vi "MatrixDUTSwitch.vi"(8 "error in (no error)":errorcluster, 10 "Channel #":string, 11 "KE3700A in":refnum<class "KE3706A.lvclass">) -> (0 "error out":errorcluster, 3 "KE3700A out":refnum<class "KE3706A.lvclass">)   [LabVIEW 2013, in "KE3706A.lvclass"]
uses:
  KE3706A.lvclass
  <instrlib>/Keithley 3706/Keithley 3700 Series.lvlib
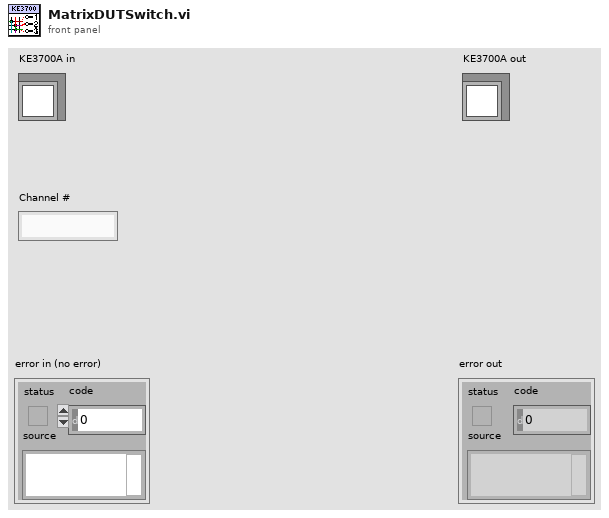
[diagram p1: front panel]
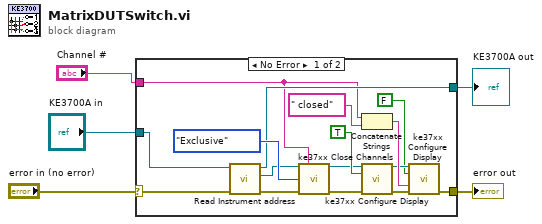
[diagram p0: block diagram]
diagram:
  n1 = case shown="No Error" "error in (no error)" {
    selector: "error in (no error)" -> [w19 w23]
    tunnel: [w7 w23] -> w4
    tunnel: "KE3700A in" -> [w20 w22]
    tunnel: [w16 w22] -> w2
    tunnel: "Channel #" -> [w6 _]
    frame No Error {
      n2 = call-dynamic "Read Instrument address.vi"("error in (no error)"=w19, "InstControl in"=w20) -> ("error out"=w18:errorcluster, "GPIB address"=w17:refnum<visa-resource-name>, "InstControl out"=w16:refnum<class "KE3706A.lvclass">)  [unwired: 7 in]
      n3 = call <instrlib>:"ke37xx Close Channels.vi"("VISA Resource Name"=w17, "Channel List"=w6, "Mode (0: Normal)"=enum16{"Normal", "Exclusive", "Slot Exclusive"}."Exclusive", "error in (no error)"=w18) -> ("VISA Resource Name Out"=w9:refnum<visa-resource-name>, "error out"=w8:errorcluster)  [unwired: 10 in]
      n4 = Concatenate Strings(w6, " closed") -> (w15:string)
      n5 = call <instrlib>:"ke37xx Configure Display.vi"("VISA Resource Name"=w9, "Clear Display (False)"=TRUE, "error in (no error)"=w8) -> ("VISA Resource Name Out"=w13:refnum<visa-resource-name>, "error out"=w10:errorcluster)  [unwired: 11 in]
      n6 = call <instrlib>:"ke37xx Configure Display.vi"("VISA Resource Name"=w13, "Clear Display (False)"=FALSE, "Message (Empty)"=w15, "error in (no error)"=w10) -> ("error out"=w7:errorcluster)  [unwired: 10 in, 1 out]
    }
    frame Error {
    }
  }
  "error out" <- w4
  "KE3700A out" <- w2
